vi "复材超声C扫缺陷分析评定软件-用于参考.vi"() -> ()   [LabVIEW 2018]
doc: "使用该模板构建用户界面事件处理设计模式。将模板应用于对话框及其它用户界面。用户也可创建并执行VI可按照与用户界面事件相同方式处理的用户定义事件。"
uses:
  <vilib>/vision/NI_Vision_Development_Module.lvlib
panel:
  out "辅助缺陷评定结果":cluster{dbl, dbl, dbl, dbl, dbl, dbl[][]}
  out "产品规格":cluster{"产品长度（周长）（mm）":dbl, "产品宽度（母线长）（mm）":dbl}
  out "Image Path":path
  out "图像分辨率":T1
  out "Source Image Pixels (U8)":u8[][](array[numeric])
  out "直方图":T2(graph)
  in  "生成原始记录":bool
  in  "去除标注信息":bool caption="缺陷评定"
  in  "缺陷分析及评定":bool caption="辅助定性分析"
  in  "缺陷测量及标注":bool caption="定量分析"
  in  "自定义色彩":bool
  in  "图像处理":bool
  out "Image":T3(plugin-control)
  in  "导入图片":bool
  in  "stop":bool caption="停止"
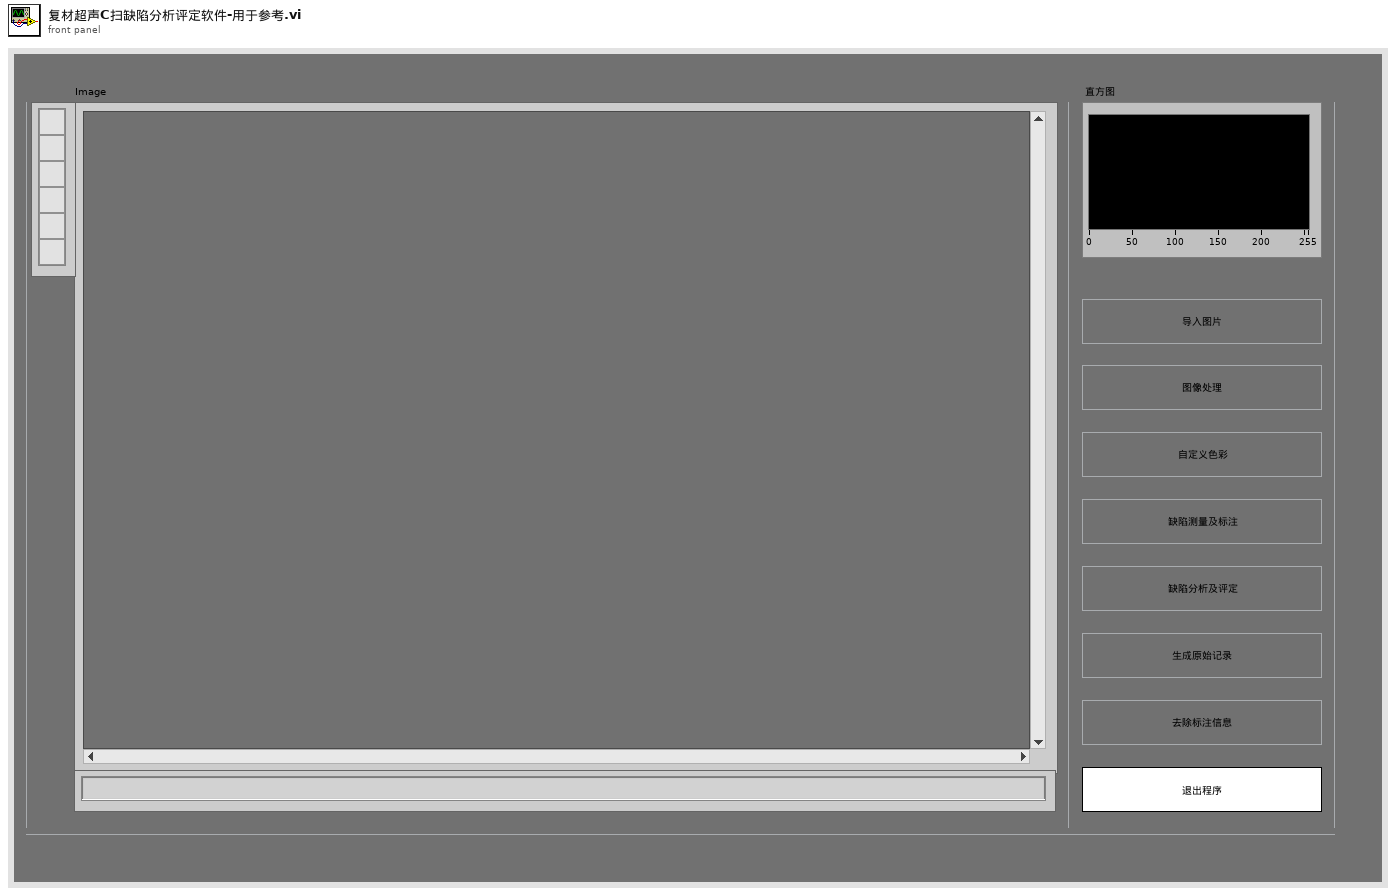
[diagram p1: front panel]
types:
  T1 = cluster{"图像X向分辨率（mm/像素）":dbl, "图像Y向分辨率（mm/像素）":dbl}
  T2 = cluster{"Starting Value":sgl, "Incremental Value":sgl, "Histogram":u32[]}
  T3 = typedef "IMAQ Image.ctl" = refnum<image>
  T4 = cluster{"Zoom Tool":bool, "Selection Tool":bool, "Pan Tool":bool, "Point Tool":bool, "Line Tool":bool, "Rectangle Tool":bool, "Rotated Rectangle Tool":bool, "Polyline Tool":bool, "Polygon Tool":bool, "Freehand Tool":bool, "Closed Freehand Tool":bool, "Ellipse Tool":bool, "Annulus Tool":bool}
  T5 = enum32{"Invalid", "Standard", "Closed", "Hidden", "Minimized", "Maximized"}
  T6 = enum32{"Linear", "Log", "Exp", "Square", "Square root", "Power X", "Power 1/X"}
  T7 = enum32{"Gray", "Binary", "Gradient", "Rainbow", "Temperature"}
  T8 = cluster{"Font Name":string, "Size":i16, "Strikeout?":bool, "Italic?":bool, "Underline?":bool, "Outline?":bool, "Shadow?":bool, "Bold?":bool, "Rotation Angle":dbl}
  T9 = cluster{"Desired Font (Application)":enum16{"User-specified Font", "Application Font", "System Font", "Dialog Font"}, "[User-specified Font]":cluster{"Font Name":string, "Size":i16, "Strikeout?":bool, "Italic?":bool, "Underline?":bool, "Outline?":bool, "Shadow?":bool, "Bold?":bool, "Rotation Angle":dbl}, "Horizontal Alignment":i16, "Vertical Alignment":i16}
  T10 = typedef "Image Type" = u32
  T11 = typedef "imagedata.ctl" = cluster{"image type":i32, "image depth":i32, "image":u8[], "mask":u8[], "colors":u32[], "Rectangle":cluster{"left":i16, "top":i16, "right":i16, "bottom":i16}}
  T12 = cluster{"Red (or Hue) value":u8, "Green (or Sat) value":u8, "Blue (or Light or Val) value":u8}[]
  T13 = typedef "IMAQ Rectangle" = cluster{"Left":i32, "Top":i32, "Right":i32, "Bottom":i32, "Rotation":dbl}
  T14 = typedef "ROI Descriptor" = cluster{"Global Rectangle":i32[], "Contours":cluster{"ID":enum32{"External", "Internal"}, "Type":u32, "Coordinates":i32[]}[]}
  T15 = cluster{"X左上":i32, "Y左上":i32, "X右上":i32, "Y右上":i32, "X左下":i32, "Y左下":i32, "X右下":i32, "Y右下":i32}
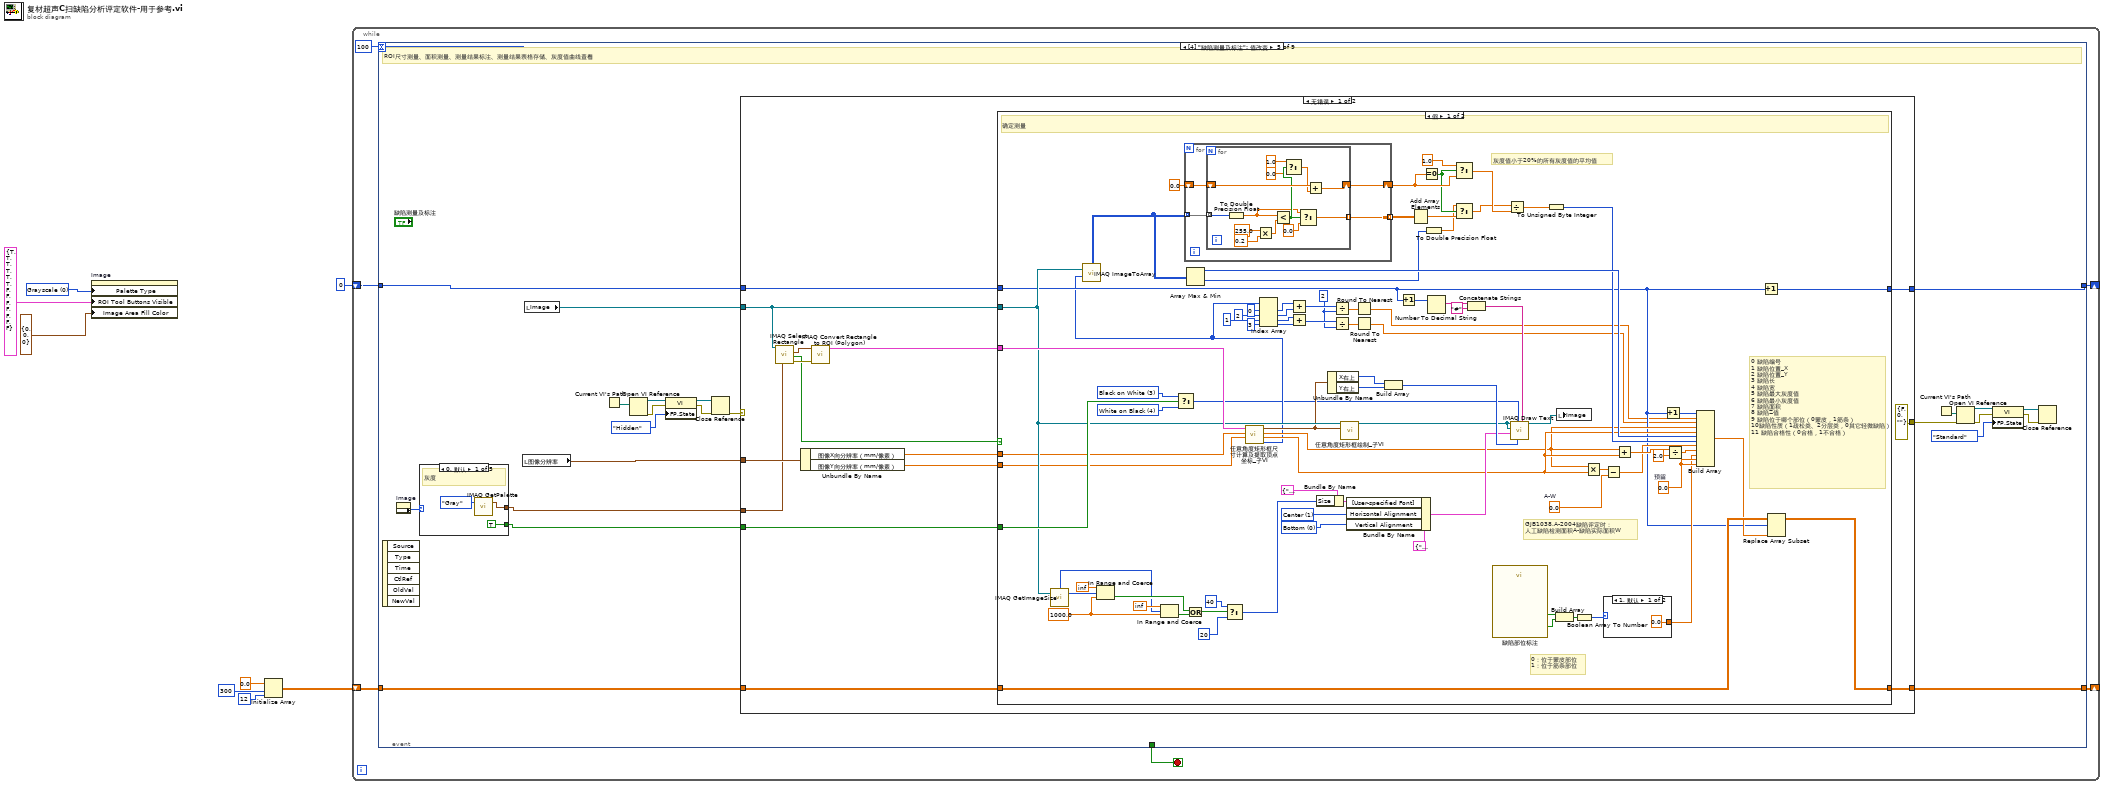
[diagram p0: block diagram]
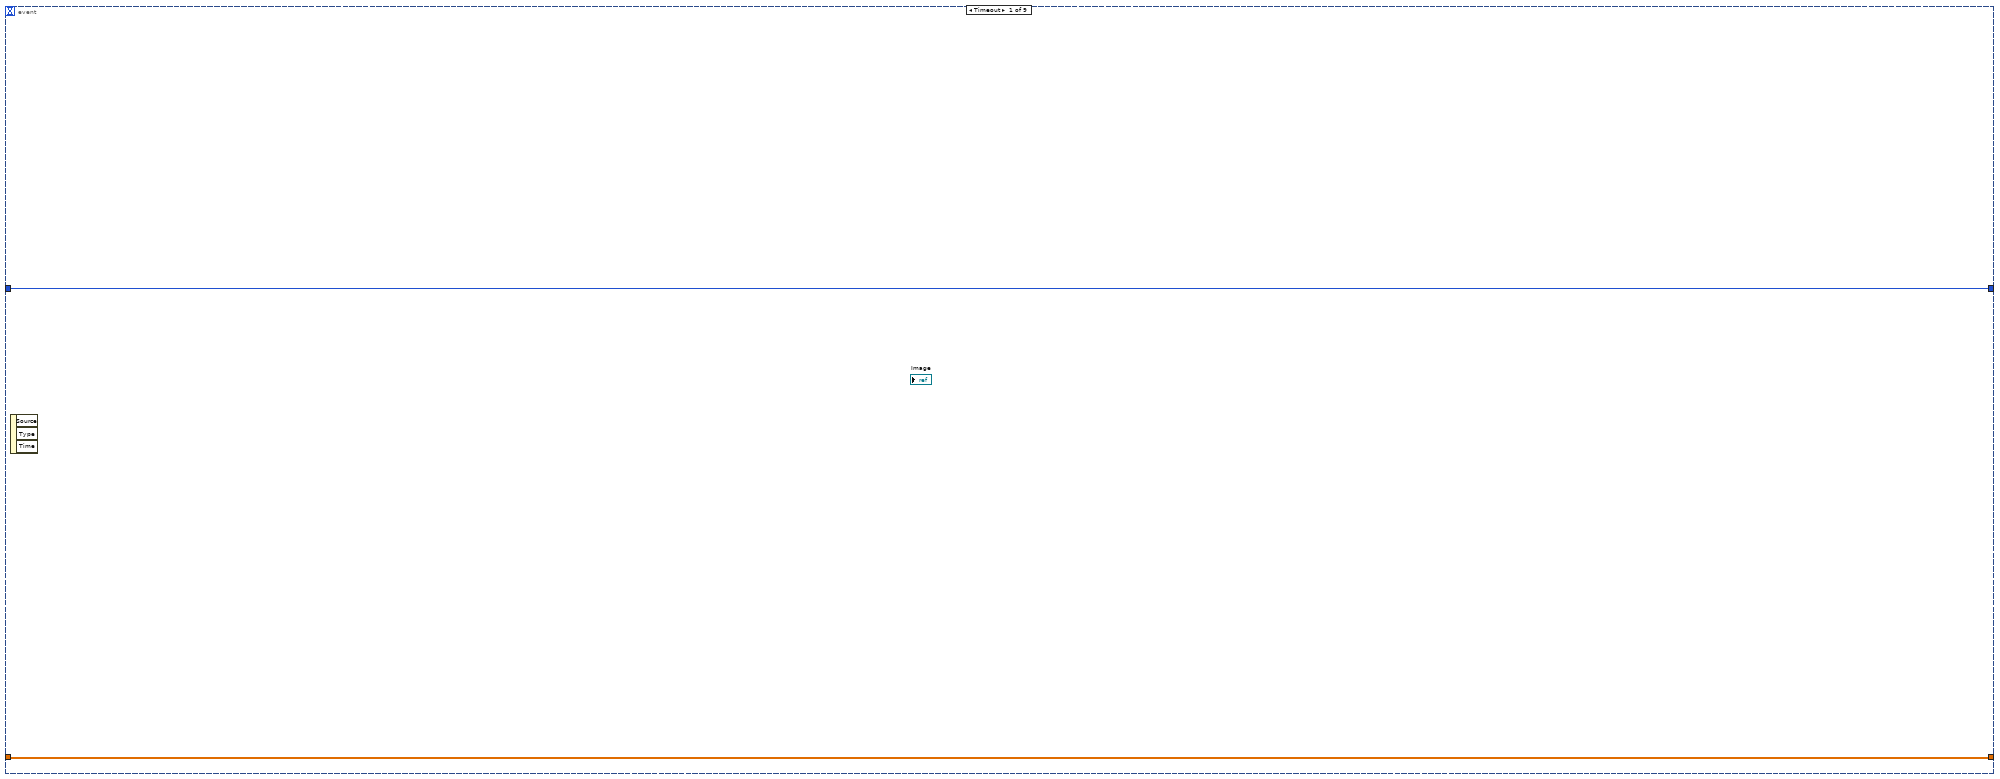
[diagram p2: hidden frame]
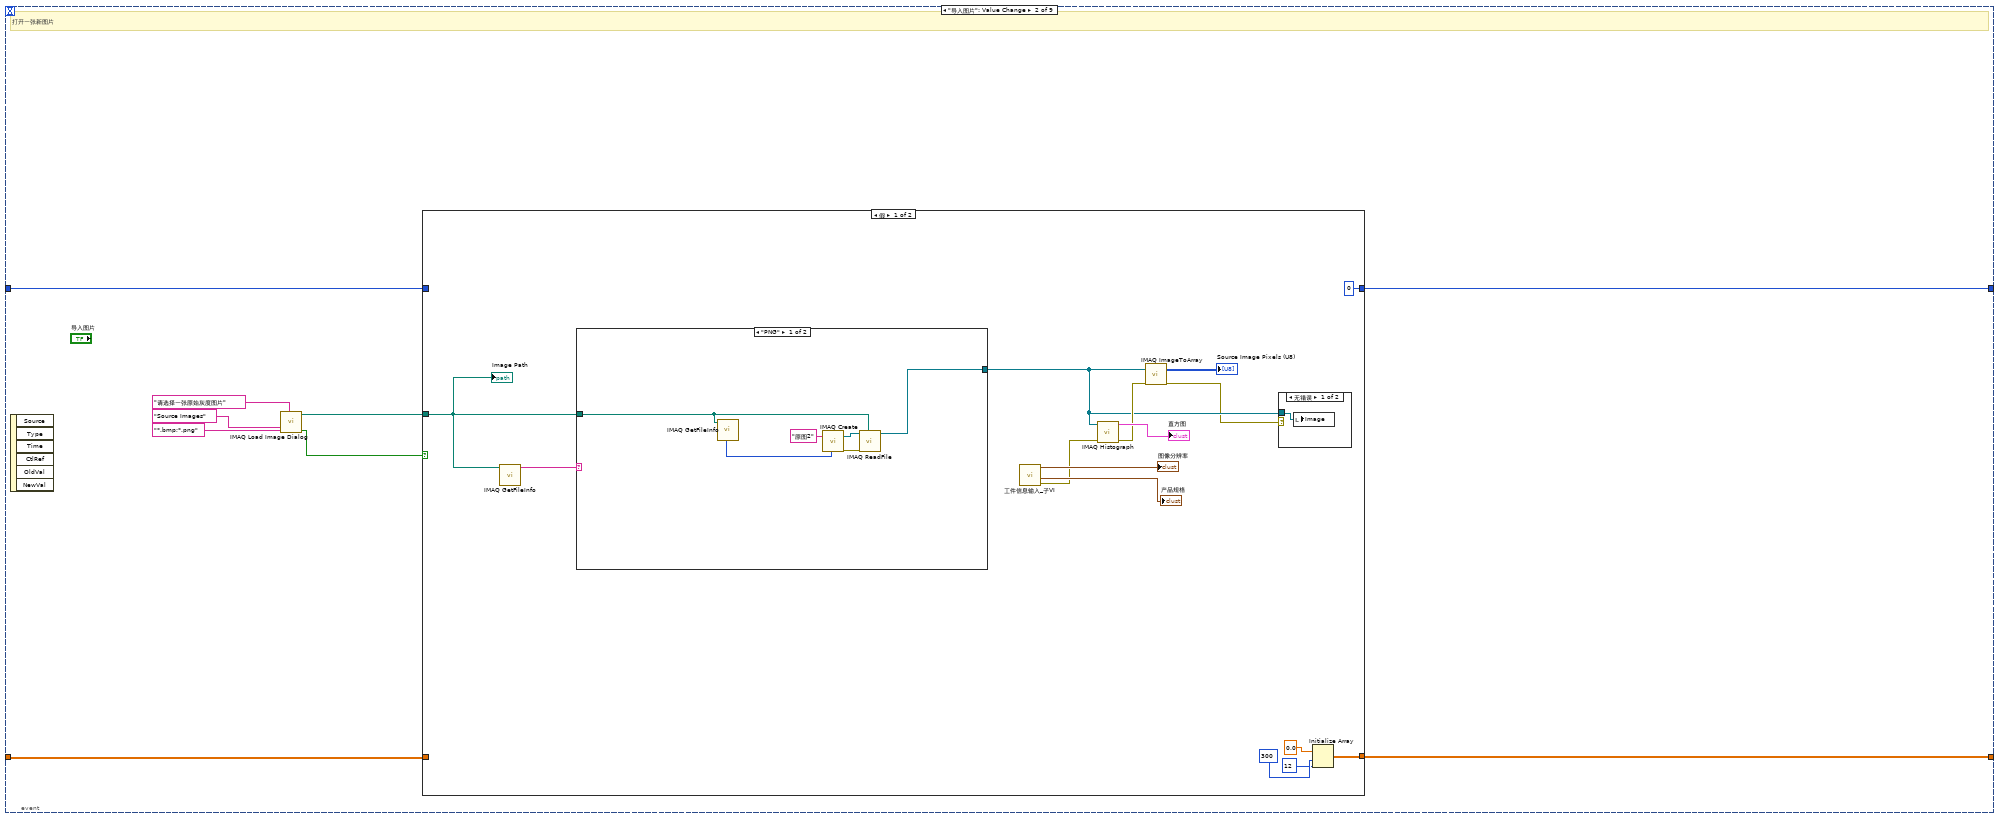
[diagram p3: hidden frame]
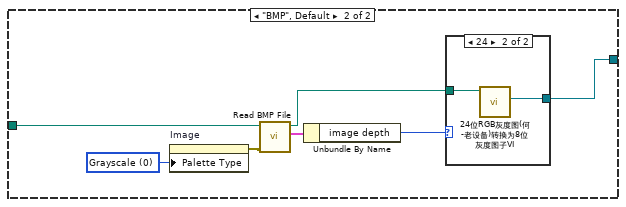
[diagram p5: hidden frame]
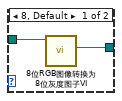
[diagram p6: hidden frame]
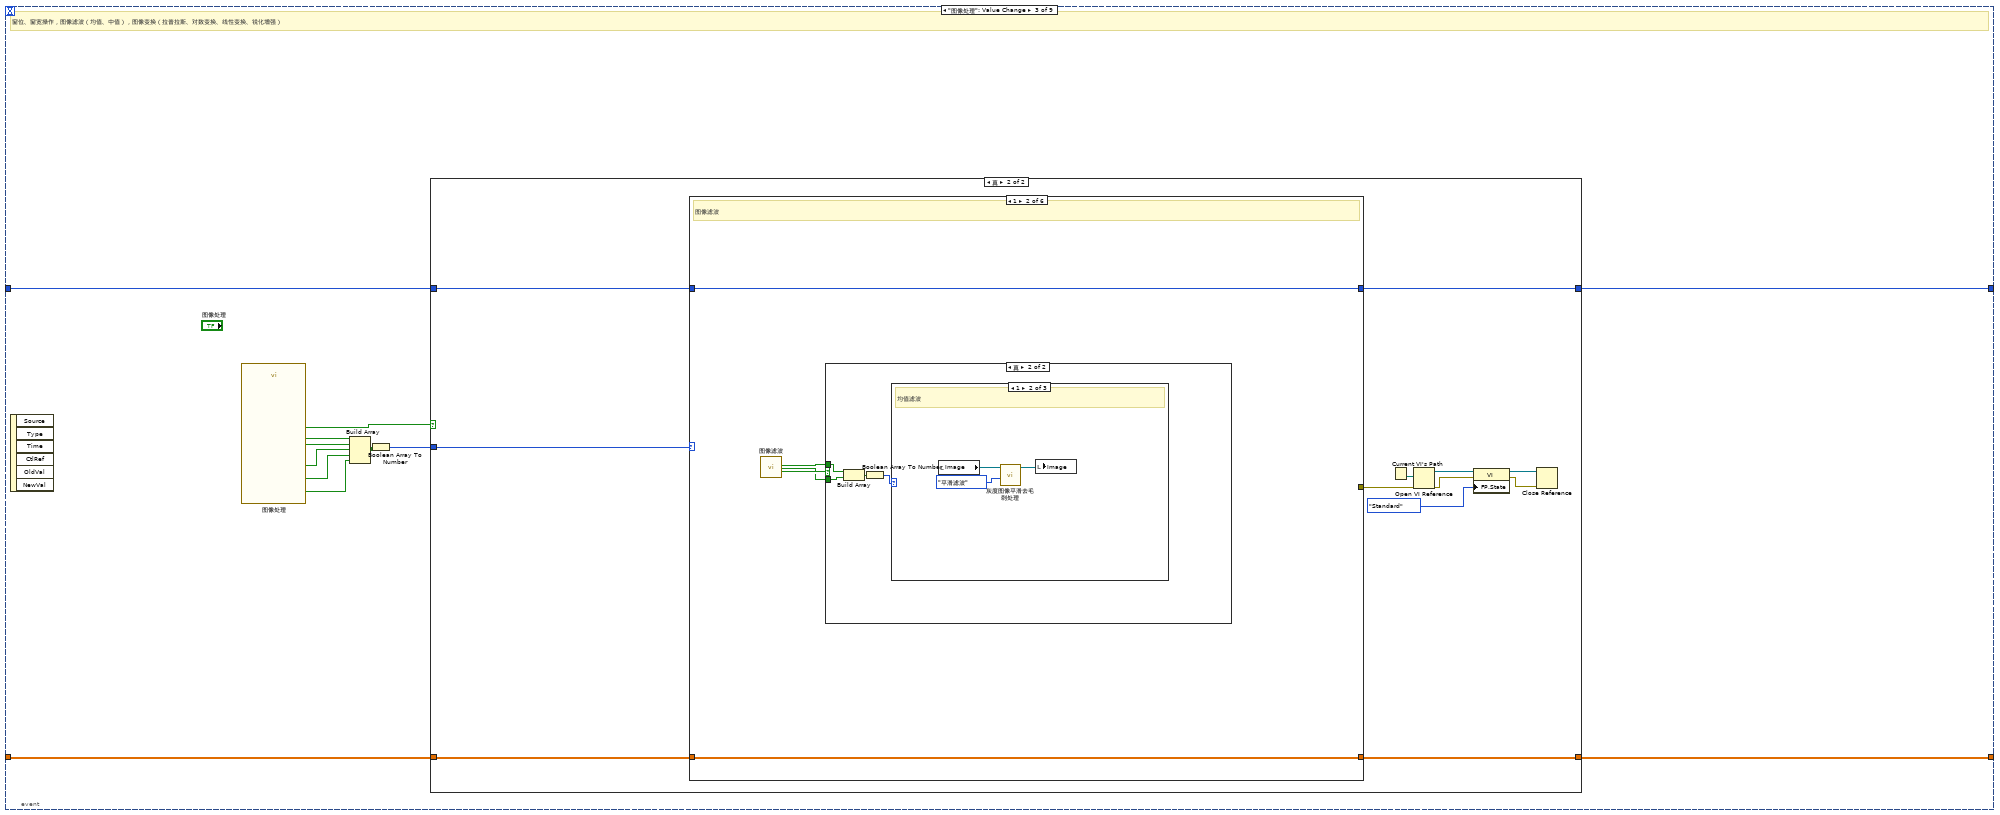
[diagram p8: hidden frame]
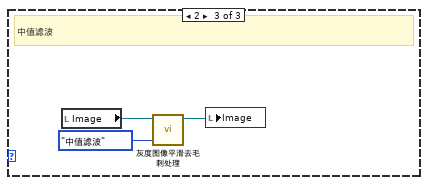
[diagram p13: hidden frame]
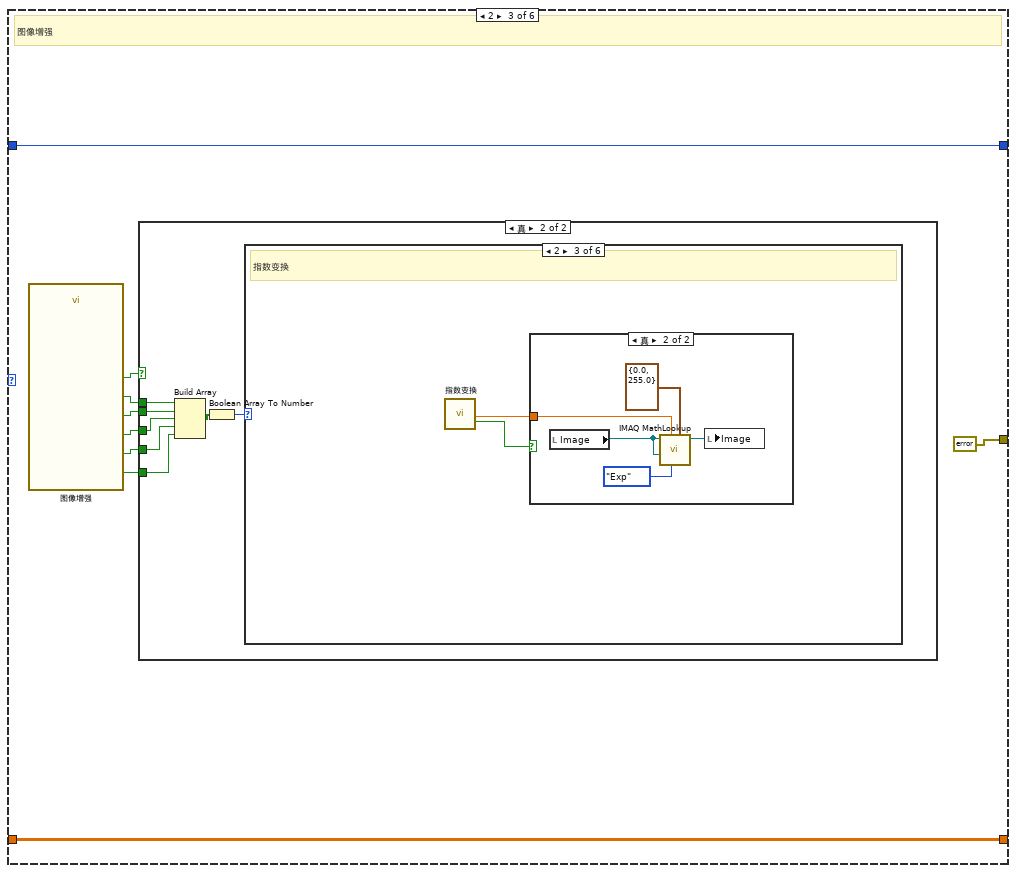
[diagram p14: hidden frame]
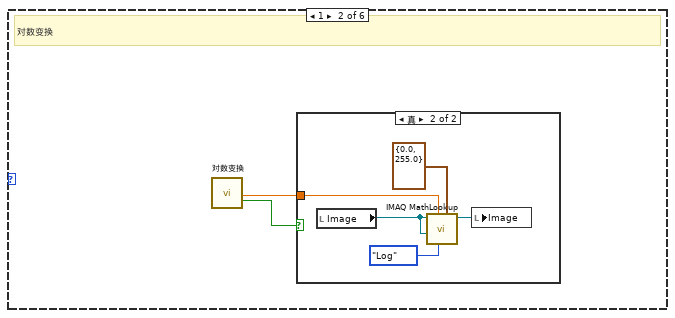
[diagram p17: hidden frame]
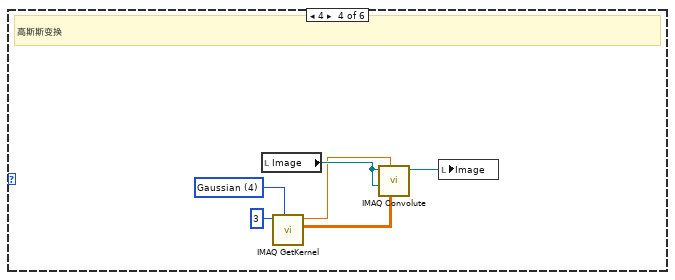
[diagram p20: hidden frame]
diagram:
  w3 = u32 0 items=["Grayscale", "Binary", "Gradient", "Rainbow", "Temperature", "User Defined", "Binary 16 Bit", "Gradient 16 Bit", "Rainbow 16 Bit", "Temperature 16 Bit", "User Defined 16 Bit"] ("Palette:Palette Type")
  n1 = property on="Image" class="ImageControl"("Palette Type"=w3, "ROI Tool Buttons Visible"=T4 {"Zoom Tool"=TRUE, "Selection Tool"=TRUE, "Pan Tool"=TRUE, "Point Tool"=TRUE, "Line Tool"=TRUE, "Rectangle Tool"=TRUE, "Rotated Rectangle Tool"=FALSE, "Polyline Tool"=FALSE, "Polygon Tool"=FALSE, "Freehand Tool"=FALSE, "Closed Freehand Tool"=FALSE, "Ellipse Tool"=FALSE, "Annulus Tool"=FALSE} ("ROI Tool Buttons Visible:All Elements"), "Image Area Fill Color"=cluster{"Red":u8, "Green":u8, "Blue":u8} {"Red"=0, "Green"=0, "Blue"=0} ("Image Area:Background:Fill Color")) -> ()  [unwired: 2 in, 2 out]
  n2 = Initialize Array(0.0 ("元素"), 300 ("维数大小"), 12 ("维数大小")) -> (w6:dbl[][])
  n3 = while {
    shift-right: [w11] -> _
    shift-left: 0 -> [w12]
    shift-right: [w10] -> _
    shift-left: w6 -> [w9]
    stop <- w14 stop-if-true
    n4 = event shown="[4] \"缺陷测量及标注\": 值改变" {
      selector: _ -> [_ _ _ _ _ _ _ _ _]
      dyn-events: _ -> [_ _ _ _ _ _ _ _ _]
      timeout: 100 -> [_ _ _ _ _ _ _ _ _]
      tunnel: [_ _ _ _ _ _ _ _ w668] -> w14
      tunnel: w12 -> [w16 w17 w64 w215 w248 w397 _ w567 _]
      tunnel: [w16 w18 w63 w215 w247 w397 0 w567 0] -> w11
      tunnel: [w15 w20 w62 w207 w246 w395 w515 w527 dbl[][] []] -> w10
      tunnel: w9 -> [w15 w19 w61 w207 w236 w396 _ w527 _]
      event Timeout {
        n5 = event-data() -> ()  [unwired: 1 in, 3 out]
      }
      event "导入图片": Value Change {
        # "打开一张新图片"
        n6 = event-data() -> ()  [unwired: 1 in, 6 out]
        n7 = call "IMAQ Load Image Dialog"("Pattern Label"="Source Images", "Prompt"="请选择一张原始灰度图片" ("prompt"), "Pattern"="*.bmp;*.png") -> ("Cancelled?"=w21:bool, "Path"=w23:path)  [unwired: 6 in, 1 out]
        n8 = case shown="假" w21 {
          tunnel: w23 -> [w35 _]
          tunnel: [w27 w60] -> w20
          tunnel: w19 -> [_ w60]
          tunnel: [0 w59] -> w18
          tunnel: w17 -> [_ w59]
          frame False {
            n9 = call "IMAQ GetFileInfo"("File Path"=w35) -> ("File Type"=w40:string)  [unwired: 4 in, 6 out]
            n10 = case shown="\"PNG\"" w40 {
              tunnel: w35 -> [w43 w54]
              tunnel: [w42 w53] -> w36
              frame "PNG" {
                n11 = call "IMAQ GetFileInfo"("File Path"=w43) -> ("Image Type"=w45:T10)  [unwired: 4 in, 6 out]
                n12 = call "IMAQ Create"("Image Name"="原图2", "Image Type"=w45) -> ("New Image"=w46:T3, "error out"=w47:errorcluster)  [unwired: 3 in]
                n13 = call "IMAQ ReadFile"("File Path"=w43, "error in (no error)"=w47, "Image"=w46) -> ("Image Out"=w42:T3)  [unwired: 4 in, 4 out]
              }
              frame "BMP", Default {
                w49 = u32 0 items=["Grayscale", "Binary", "Gradient", "Rainbow", "Temperature", "User Defined", "Binary 16 Bit", "Gradient 16 Bit", "Rainbow 16 Bit", "Temperature 16 Bit", "User Defined 16 Bit"] ("Palette:Palette Type")
                n14 = property on="Image" class="ImageControl"("Palette Type"=w49) -> (error out=w48:errorcluster)  [unwired: 2 in, 1 out]
                n15 = call <vilib>:"Read BMP File.vi"("error in (no error)"=w48, "path to BMP file"=w54) -> ("image data"=w52:T11, "path"=w50:path)  [unwired: 7 in, 1 out]
                n16 = Unbundle By Name(w52) -> ("image depth"=w51:i32)
                n17 = case shown="24" w51 {
                  tunnel: w50 -> [w56 w58]
                  tunnel: [w55 w57] -> w53
                  frame 8, Default {
                    n18 = call "8位RGB图像转换为8位灰度图子VI.vi"("path to BMP file"=w56) -> ("转换后的原始图像"=w55:T3)  [unwired: 8 in, 2 out]
                  }
                  frame 24 {
                    n19 = call "24位RGB灰度图(何-老设备)转换为8位灰度图子VI.vi"("File Path"=w58) -> ("转换后的原始图像"=w57:T3)  [unwired: 8 in, 2 out]
                  }
                }
              }
            }
            n20 = call "工件信息输入_子VI.vi"() -> ("错误常量out"=w31:errorcluster, "产品规格"=→"产品规格":cluster{"产品长度（周长）（mm）":dbl, "产品宽度（母线长）（mm）":dbl}, "图像分辨率"=→"图像分辨率":T1)  [unwired: 9 in]
            n21 = call "IMAQ Histograph"("error in (no error)"=w31, "Image"=w36) -> ("error out"=w37:errorcluster, "Histogram Graph"=→"直方图":T2)  [unwired: 6 in, 2 out]
            n22 = call "IMAQ ImageToArray"("error in (no error)"=w37, "Image"=w36) -> ("error out"=w34:errorcluster, "Image Pixels (U8)"=→"Source Image Pixels (U8)":u8[][])  [unwired: 2 in, 3 out]
            n23 = case shown="无错误" w34 {
              tunnel: w36 -> [w41 _]
              frame No Error {
                n24 = local write "Image"(w41) -> ()
              }
              frame Error {
              }
            }
            n25 = Initialize Array(0.0 ("元素"), 300 ("维数大小"), 12 ("维数大小")) -> (w27:dbl[][])
            "Image Path" <- w35
          }
          frame True {
          }
        }
      }
      event "图像处理": Value Change {
        # "窗位、窗宽操作，图像滤波（均值、中值），图像变换（拉普拉斯、对数变换、线性变换、锐化增强）"
        n26 = event-data() -> ()  [unwired: 1 in, 6 out]
        n27 = call "图像处理"() -> ("撤销图像处理"=w65:bool, "线性灰度值测量"=w66:bool, "窗位窗宽"=w71:bool, "图像增强"=w67:bool, "图像滤波"=w72:bool, "确定"=w68:bool)  [unwired: 13 in, 1 out]
        n28 = Build Array(w72, w67, w71, w66, w65) -> (w70:bool[])
        n29 = Boolean Array To Number(Boolean array=w70) -> (number=w69:u32)
        n30 = case shown="真" w68 {
          tunnel: w69 -> [_ w86]
          tunnel: w64 -> [w73 w78]
          tunnel: [w73 w77] -> w63
          tunnel: [w74 w76] -> w62
          tunnel: w61 -> [w74 w75]
          frame False {
          }
          frame True {
            n31 = case shown="1" w86 {
              tunnel: [_ _ errorcluster {"status"=FALSE, "code"=0, "source"=""} ("错误输入（无错误）") _ _ _] -> w79
              tunnel: w78 -> [w88 w89 w105 w155 w180 w201]
              tunnel: [w88 w89 w105 w155 w180 w201] -> w77
              tunnel: [w87 w90 w104 w154 w179 w202] -> w76
              tunnel: w75 -> [w87 w90 w104 w154 w179 w202]
              frame 0, Default {
              }
              frame 1 {
                # "图像滤波"
                n32 = call "图像滤波"() -> ("均值滤波"=w92:bool, "中值滤波"=w91:bool, "确定"=w93:bool)  [unwired: 16 in, 1 out]
                n33 = case shown="真" w93 {
                  tunnel: w92 -> [_ w96]
                  tunnel: w91 -> [_ w95]
                  frame False {
                  }
                  frame True {
                    n34 = Build Array(w96, w95) -> (w97:bool[])
                    n35 = Boolean Array To Number(Boolean array=w97) -> (number=w94:u32)
                    n36 = case shown="1" w94 {
                      frame 0, Default {
                      }
                      frame 1 {
                        # "均值滤波"
                        n37 = local read "Image"() -> (w100:T3)
                        n38 = call "灰度图像平滑去毛刺处理.vi"("滤波方法选择"=enum16{"中值滤波", "平滑滤波"}."平滑滤波", "Image"=w100) -> ("Image Out"=w99:T3)  [unwired: 9 in]
                        n39 = local write "Image"(w99) -> ()
                      }
                      frame 2 {
                        # "中值滤波"
                        n40 = local read "Image"() -> (w103:T3)
                        n41 = call "灰度图像平滑去毛刺处理.vi"("滤波方法选择"=enum16{"中值滤波", "平滑滤波"}."中值滤波", "Image"=w103) -> ("Image Out"=w102:T3)  [unwired: 9 in]
                        n42 = local write "Image"(w102) -> ()
                      }
                    }
                  }
                }
              }
              frame 2 {
                # "图像增强"
                n43 = call "图像增强"() -> ("幂变换"=w107:bool, "阈值变换"=w108:bool, "高斯变换"=w109:bool, "指数变换"=w110:bool, "对数变换"=w111:bool, "确定"=w112:bool)  [unwired: 13 in, 1 out]
                n44 = case shown="真" w112 {
                  tunnel: w111 -> [_ w117]
                  tunnel: w110 -> [_ w116]
                  tunnel: w109 -> [_ w115]
                  tunnel: w108 -> [_ w114]
                  tunnel: w107 -> [_ w113]
                  frame False {
                  }
                  frame True {
                    n45 = Build Array(w117, w116, w115, w114, w113) -> (w119:bool[])
                    n46 = Boolean Array To Number(Boolean array=w119) -> (number=w118:u32)
                    n47 = case shown="2" w118 {
                      frame 0, Default {
                      }
                      frame 1 {
                        # "对数变换"
                        n48 = call "对数变换"() -> ("变换系数K"=w120:dbl, "确定"=w121:bool)  [unwired: 17 in, 1 out]
                        n49 = case shown="真" w121 {
                          tunnel: w120 -> [_ w122]
                          frame False {
                          }
                          frame True {
                            n50 = local read "Image"() -> (w126:T3)
                            n51 = call "IMAQ MathLookup"("Range"=cluster{"Minimum":sgl, "Maximum":sgl} {"Minimum"=0.0, "Maximum"=255.0}, "Operator"=T6."Log", "X Value"=w122, "Image Dst"=w126, "Image Src"=w126) -> ("Image Dst Out"=w124:T3)  [unwired: 5 in, 1 out]
                            n52 = local write "Image"(w124) -> ()
                          }
                        }
                      }
                      frame 2 {
                        # "指数变换"
                        n53 = call "指数变换"() -> ("变换系数K"=w127:dbl, "确定"=w128:bool)  [unwired: 17 in, 1 out]
                        n54 = case shown="真" w128 {
                          tunnel: w127 -> [_ w129]
                          frame False {
                          }
                          frame True {
                            n55 = local read "Image"() -> (w133:T3)
                            n56 = call "IMAQ MathLookup"("Range"=cluster{"Minimum":sgl, "Maximum":sgl} {"Minimum"=0.0, "Maximum"=255.0}, "Operator"=T6."Exp", "X Value"=w129, "Image Dst"=w133, "Image Src"=w133) -> ("Image Dst Out"=w131:T3)  [unwired: 5 in, 1 out]
                            n57 = local write "Image"(w131) -> ()
                          }
                        }
                      }
                      frame 4 {
                        w139 = u16 4 items=["Gradient"=1, "Laplacian"=2, "Smoothing"=3, "Gaussian"=4] ("Kernel Family")
                        # "高斯斯变换"
                        n58 = local read "Image"() -> (w136:T3)
                        n59 = call "IMAQ GetKernel"("Kernel Family"=w139, "Kernel Size (3,5,...)"=3) -> ("Kernel"=w137:sgl[][], "Divider"=w134:sgl)  [unwired: 6 in, 2 out]
                        n60 = call "IMAQ Convolute"("Kernel"=w137, "Divider (kernel sum)"=w134, "Image Dst"=w136, "Image Src"=w136) -> ("Image Dst Out"=w135:T3)  [unwired: 6 in, 1 out]
                        n61 = local write "Image"(w135) -> ()
                      }
                      frame 8 {
                        # "阈值变换"
                        n62 = call "阈值范围选择子VI.vi"() -> ("阈值范围"=w140:cluster{"Lower value":sgl, "Upper value":sgl}, "确定执行"=w141:bool)  [unwired: 10 in]
                        n63 = case shown="真" w141 {
                          tunnel: w140 -> [_ w143]
                          frame False {
                          }
                          frame True {
                            n64 = local read "Image"() -> (w146:T3)
                            n65 = call "IMAQ Threshold"("Replace Value"=sgl 255.0, "Keep/Replace Value (Replace)"=TRUE, "Range"=w143, "Image Dst"=w146, "Image Src"=w146) -> ("Image Dst Out"=w145:T3)  [unwired: 5 in, 1 out]
                            n66 = local write "Image"(w145) -> ()
                          }
                        }
                      }
                      frame 16 {
                        # "幂变换"
                        n67 = call "幂变换"() -> ("变换系数K"=w147:dbl, "确定"=w148:bool)  [unwired: 17 in, 1 out]
                        n68 = case shown="真" w148 {
                          tunnel: w147 -> [_ w149]
                          frame False {
                          }
                          frame True {
                            n69 = local read "Image"() -> (w153:T3)
                            n70 = call "IMAQ MathLookup"("Range"=cluster{"Minimum":sgl, "Maximum":sgl} {"Minimum"=0.0, "Maximum"=255.0}, "Operator"=T6."Power 1/X", "X Value"=w149, "Image Dst"=w153, "Image Src"=w153) -> ("Image Dst Out"=w151:T3)  [unwired: 5 in, 1 out]
                            n71 = local write "Image"(w151) -> ()
                          }
                        }
                      }
                    }
                  }
                }
              }
              frame 4 {
                # "窗位窗宽"
                n72 = Two Button Dialog(message="确定进行窗位窗宽操作？" ("消息")) -> (T button?=w157:bool)  [unwired: 2 in]
                n73 = case shown="真" w157 {
                  frame False {
                  }
                  frame True {
                    n74 = property on="Image" class="ImageControl"() -> (error out=w159:errorcluster, "Palette Type"=w166:u32)  [unwired: 2 in, 1 out]
                    n75 = Current VI's Path() -> (path=w161:path)
                    n76 = Open VI Reference(vi path=w161, error in (no error)=w159) -> (vi reference=w162:refnum<vi>, error out=w164:errorcluster)  [unwired: 4 in]
                    n77 = case shown="4" w166 {
                      tunnel: [w170 w172 w174 w176 w178] -> w167
                      frame 0, Default {
                        # "灰度"
                        n78 = call "IMAQ GetPalette"("Palette Number (gray)"=T7."Gray") -> ("Color Palette"=w170:cluster{"Red":u8, "Green":u8, "Blue":u8}[])  [unwired: 4 in, 1 out]
                      }
                      frame 2 {
                        # "梯度"
                        n79 = call "IMAQ GetPalette"("Palette Number (gray)"=T7."Gradient") -> ("Color Palette"=w172:cluster{"Red":u8, "Green":u8, "Blue":u8}[])  [unwired: 4 in, 1 out]
                      }
                      frame 3 {
                        # "彩虹"
                        n80 = call "IMAQ GetPalette"("Palette Number (gray)"=T7."Rainbow") -> ("Color Palette"=w174:cluster{"Red":u8, "Green":u8, "Blue":u8}[])  [unwired: 4 in, 1 out]
                      }
                      frame 4 {
                        # "温度"
                        n81 = call "IMAQ GetPalette"("Palette Number (gray)"=T7."Temperature") -> ("Color Palette"=w176:cluster{"Red":u8, "Green":u8, "Blue":u8}[])  [unwired: 4 in, 1 out]
                      }
                      frame 5 {
                        # "自定义"
                        n82 = property on="Image" class="ImageControl"() -> ("User Palette"=w178:cluster{"Red":u8, "Green":u8, "Blue":u8}[])  [unwired: 2 in, 2 out]
                      }
                    }
                    n83 = property class="VI"(reference=w162, error in=w164, "FP.State"=T5."Hidden" ("前面板窗口:状态")) -> (reference out=w163:refnum<vi>, error out=w165:errorcluster)
                    n84 = local read "Source Image Pixels (U8)"() -> (w168:u8[][])
                    n85 = Close Reference(reference=w163, error in (no error)=w165) -> ()  [unwired: 1 out]
                    n86 = local read "Image"() -> (w158:T3)
                    n87 = call "窗位窗宽调整子VI.vi"("Image in"=w158, "Palette:User Palette"=w167, "Palette:Palette Type"=w166, "Image Pixels (U8)"=w168) -> ("Image out"=w169:T3)  [unwired: 7 in]
                    n88 = local write "Image"(w169) -> ()
                  }
                }
              }
              frame 8 {
                # "查看线灰度值曲线，用于精确测量"
                n89 = Current VI's Path() -> (path=w187:path)
                n90 = Open VI Reference(vi path=w187) -> (vi reference=w186:refnum<vi>, error out=w184:errorcluster)  [unwired: 5 in]
                n91 = property class="VI"(reference=w186, error in=w184, "FP.State"=T5."Hidden" ("前面板窗口:状态")) -> (reference out=w185:refnum<vi>, error out=w183:errorcluster)
                n92 = Close Reference(reference=w185, error in (no error)=w183) -> (error out=w181:errorcluster)
                n93 = case shown="无错误" w181 {
                  frame No Error {
                    n94 = property on="Image" class="ImageControl"() -> ("Palette Type"=w189:u32)  [unwired: 2 in, 2 out]
                    n95 = case shown="2" w189 {
                      tunnel: [w192 w194 w196 w198 w200] -> w188
                      frame 0, Default {
                        # "灰度"
                        n96 = call "IMAQ GetPalette"("Palette Number (gray)"=T7."Gray") -> ("Color Palette"=w192:cluster{"Red":u8, "Green":u8, "Blue":u8}[])  [unwired: 4 in, 1 out]
                      }
                      frame 2 {
                        # "梯度"
                        n97 = call "IMAQ GetPalette"("Palette Number (gray)"=T7."Gradient") -> ("Color Palette"=w194:cluster{"Red":u8, "Green":u8, "Blue":u8}[])  [unwired: 4 in, 1 out]
                      }
                      frame 3 {
                        # "彩虹"
                        n98 = call "IMAQ GetPalette"("Palette Number (gray)"=T7."Rainbow") -> ("Color Palette"=w196:cluster{"Red":u8, "Green":u8, "Blue":u8}[])  [unwired: 4 in, 1 out]
                      }
                      frame 4 {
                        # "温度"
                        n99 = call "IMAQ GetPalette"("Palette Number (gray)"=T7."Temperature") -> ("Color Palette"=w198:cluster{"Red":u8, "Green":u8, "Blue":u8}[])  [unwired: 4 in, 1 out]
                      }
                      frame 5 {
                        # "自定义"
                        n100 = property on="Image" class="ImageControl"() -> ("User Palette"=w200:cluster{"Red":u8, "Green":u8, "Blue":u8}[])  [unwired: 2 in, 2 out]
                      }
                    }
                    n101 = local read "Image"() -> (w191:T3)
                    n102 = local read "图像分辨率"() -> (w190:T1)
                    n103 = call "线性灰度值曲线查看子VI.vi"("Palette:User Palette"=w188, "图像分辨率"=w190, "Image"=w191) -> ()  [unwired: 9 in]
                  }
                  frame Error {
                  }
                }
              }
              frame 16 {
                # "撤销图像处理，恢复原图"
                n104 = local read "Source Image Pixels (U8)"() -> (w206:u8[][])
                n105 = call "IMAQ Create"("Image Name"="P1") -> ("New Image"=w205:T3)  [unwired: 4 in, 1 out]
                n106 = call "IMAQ ArrayToImage"("Image Pixels (U8)"=w206, "Image"=w205) -> ("Image Out"=w204:T3)  [unwired: 8 in, 1 out]
                n107 = local write "Image"(w204) -> ()
              }
            }
            n108 = Current VI's Path() -> (path=w85:path)
            n109 = Open VI Reference(vi path=w85, error in (no error)=w79) -> (vi reference=w84:refnum<vi>, error out=w81:errorcluster)  [unwired: 4 in]
            n110 = property class="VI"(reference=w84, error in=w81, "FP.State"=T5."Standard" ("前面板窗口:状态")) -> (reference out=w82:refnum<vi>, error out=w80:errorcluster)
            n111 = Close Reference(reference=w82, error in (no error)=w80) -> ()  [unwired: 1 out]
          }
        }
      }
      event "自定义色彩": Value Change {
        # "色彩、色阶自定义"
        n112 = event-data() -> ()  [unwired: 1 in, 6 out]
        n113 = call "调色板"() -> ("自定义显示"=w209:bool, "温度显示"=w210:bool, "彩虹显示"=w211:bool, "梯度显示"=w212:bool, "灰度显示"=w213:bool, "确定"=w214:bool)  [unwired: 13 in, 1 out]
        n114 = Build Array(w213, w212, w211, w210, w209) -> (w208:bool[])
        n115 = case shown="真" w214 {
          tunnel: w208 -> [_ w218]
          frame False {
          }
          frame True {
            n116 = Boolean Array To Number(Boolean array=w218) -> (number=w217:u32)
            n117 = case shown="16" w217 {
              tunnel: [w219 w220 w221 w222 w223 w225] -> w216
              frame 0, Default {
                w219 = u32 0 items=["Grayscale", "Binary", "Gradient", "Rainbow", "Temperature", "User Defined", "Binary 16 Bit", "Gradient 16 Bit", "Rainbow 16 Bit", "Temperature 16 Bit", "User Defined 16 Bit"] ("Palette:Palette Type")
              }
              frame 1 {
                w220 = u32 0 items=["Grayscale", "Binary", "Gradient", "Rainbow", "Temperature", "User Defined", "Binary 16 Bit", "Gradient 16 Bit", "Rainbow 16 Bit", "Temperature 16 Bit", "User Defined 16 Bit"] ("Palette:Palette Type")
                # "灰度"
              }
              frame 2 {
                w221 = u32 2 items=["Grayscale", "Binary", "Gradient", "Rainbow", "Temperature", "User Defined", "Binary 16 Bit", "Gradient 16 Bit", "Rainbow 16 Bit", "Temperature 16 Bit", "User Defined 16 Bit"] ("Palette:Palette Type")
                # "梯度"
              }
              frame 4 {
                w222 = u32 3 items=["Grayscale", "Binary", "Gradient", "Rainbow", "Temperature", "User Defined", "Binary 16 Bit", "Gradient 16 Bit", "Rainbow 16 Bit", "Temperature 16 Bit", "User Defined 16 Bit"] ("Palette:Palette Type")
                # "彩虹"
              }
              frame 8 {
                w223 = u32 4 items=["Grayscale", "Binary", "Gradient", "Rainbow", "Temperature", "User Defined", "Binary 16 Bit", "Gradient 16 Bit", "Rainbow 16 Bit", "Temperature 16 Bit", "User Defined 16 Bit"] ("Palette:Palette Type")
                # "温度"
              }
              frame 16 {
                w225 = u32 5 items=["Grayscale", "Binary", "Gradient", "Rainbow", "Temperature", "User Defined", "Binary 16 Bit", "Gradient 16 Bit", "Rainbow 16 Bit", "Temperature 16 Bit", "User Defined 16 Bit"] ("Palette:Palette Type")
                # "自定义"
                n118 = call "自定义成像色谱20200214.vi"() -> ("Color palette"=w224:T12)  [unwired: 8 in, 1 out]
                n119 = property on="Image" class="ImageControl"("User Palette"=w224) -> ()  [unwired: 2 in, 2 out]
              }
            }
            n120 = property on="Image" class="ImageControl"("Palette Type"=w216) -> ()  [unwired: 2 in, 2 out]
          }
        }
      }
      event "缺陷测量及标注": Value Change {
        # "ROI尺寸测量、面积测量、测量结果标注、测量结果表格存储、灰度值曲线查看"
        n121 = event-data() -> ()  [unwired: 1 in, 6 out]
        n122 = property on="Image" class="ImageControl"() -> ("Palette Type"=w245:u32)  [unwired: 2 in, 2 out]
        n123 = case shown="0, 默认" w245 {
          tunnel: [w373 w375 w377 w379 w381] -> w244
          tunnel: [TRUE _ _ _ _] -> w237
          frame 0, Default {
            # "灰度"
            n124 = call "IMAQ GetPalette"("Palette Number (gray)"=T7."Gray") -> ("Color Palette"=w373:cluster{"Red":u8, "Green":u8, "Blue":u8}[])  [unwired: 4 in, 1 out]
          }
          frame 2 {
            # "梯度"
            n125 = call "IMAQ GetPalette"("Palette Number (gray)"=T7."Gradient") -> ("Color Palette"=w375:cluster{"Red":u8, "Green":u8, "Blue":u8}[])  [unwired: 4 in, 1 out]
          }
          frame 3 {
            # "彩虹"
            n126 = call "IMAQ GetPalette"("Palette Number (gray)"=T7."Rainbow") -> ("Color Palette"=w377:cluster{"Red":u8, "Green":u8, "Blue":u8}[])  [unwired: 4 in, 1 out]
          }
          frame 4 {
            # "温度"
            n127 = call "IMAQ GetPalette"("Palette Number (gray)"=T7."Temperature") -> ("Color Palette"=w379:cluster{"Red":u8, "Green":u8, "Blue":u8}[])  [unwired: 4 in, 1 out]
          }
          frame 5 {
            # "自定义"
            n128 = property on="Image" class="ImageControl"() -> ("User Palette"=w381:cluster{"Red":u8, "Green":u8, "Blue":u8}[])  [unwired: 2 in, 2 out]
          }
        }
        n129 = local read "图像分辨率"() -> (w234:T1)
        n130 = local read "Image"() -> (w235:T3)
        n131 = Current VI's Path() -> (path=w233:path)
        n132 = Open VI Reference(vi path=w233) -> (vi reference=w232:refnum<vi>, error out=w230:errorcluster)  [unwired: 5 in]
        n133 = property class="VI"(reference=w232, error in=w230, "FP.State"=T5."Hidden" ("前面板窗口:状态")) -> (reference out=w231:refnum<vi>, error out=w229:errorcluster)
        n134 = Close Reference(reference=w231, error in (no error)=w229) -> (error out=w227:errorcluster)
        n135 = case shown="无错误" w227 {
          tunnel: w248 -> [w263 w370]
          tunnel: [w262 w370] -> w247
          tunnel: w235 -> [w253 _]
          tunnel: w234 -> [w261 _]
          tunnel: [w260 w371] -> w246
          tunnel: w236 -> [w259 w371]
          tunnel: w244 -> [w252 _]
          tunnel: w237 -> [w258 _]
          tunnel: [errorcluster {"status"=FALSE, "code"=0, "source"=""} ("error in (no error)") _] -> w226
          frame No Error {
            n136 = call "IMAQ Select Rectangle"("Color Palette"=w252, "Image In"=w253) -> ("error out"=w254:errorcluster, "Cancelled"=w249:bool, "Rectangle"=w255:T13)  [unwired: 6 in, 1 out]
            n137 = Unbundle By Name(w261) -> ("图像X向分辨率（mm/像素）"=w257:dbl, "图像Y向分辨率（mm/像素）"=w256:dbl)
            n138 = call "IMAQ Convert Rectangle to ROI (Polygon)"("error in (no error)"=w254, "Rectangle"=w255) -> ("ROI Descriptor"=w251:T14)  [unwired: 6 in, 2 out]
            n139 = case shown="假" w249 {
              tunnel: w263 -> [w292 w369]
              tunnel: [w348 w369] -> w262
              tunnel: w253 -> [w301 _]
              tunnel: [w340 w368] -> w260
              tunnel: w259 -> [w342 w368]
              tunnel: w251 -> [w302 _]
              tunnel: w258 -> [w314 _]
              tunnel: w257 -> [w300 _]
              tunnel: w256 -> [w299 _]
              frame False {
                w272 = 2 ("y")
                w290 = i16 0 items=["Bottom", "Top", "Baseline"] ("Vertical Alignment")
                w288 = 1000.0 ("下限")
                w312 = 4 items=["White", "Black", "Inverted", "Black on White", "White on Black"] ("Color")
                w328 = 0.0  # A-W
                w336 = 0.0  # 预留
                w313 = 3 items=["White", "Black", "Inverted", "Black on White", "White on Black"] ("Color")
                w291 = i16 1 items=["Left", "Center", "Right"] ("Horizontal Alignment")
                # "灰度值小于20%的所有灰度值的平均值"
                # "GJB1038.A-2004缺陷评定时：\n人工缺陷检测面积A-缺陷实际面积W"
                # "0：位于蒙皮部位\n1：位于筋条部位"
                # "0 缺陷编号\n1 缺陷位置_X\n2 缺陷位置_Y\n3 缺陷长\n4 缺陷宽\n5 缺陷最大灰度值\n6 缺陷最小灰度值\n7 缺陷面积\n8 缺陷Z值\n9 缺陷位于哪个部位（0蒙皮，1筋条）\n10缺陷性质（1疏松类、2分层类，0其它轻微缺陷）\n11 缺陷合格性（0合格，1不合格）"
                # "确定测量"
                n140 = call "IMAQ GetImageSize"("Image"=w301) -> ("Y Resolution"=w307:i32, "X Resolution"=w306:i32)  [unwired: 3 in, 1 out]
                n141 = In Range and Coerce(upper limit=inf, x=w307, lower limit=w288) -> (In Range?=w309:bool)  [unwired: 1 out]
                n142 = In Range and Coerce(upper limit=inf, x=w306, lower limit=w288) -> (In Range?=w308:bool)  [unwired: 1 out]
                n143 = Select(t=w313, s=w314, f=w312) -> (s? t:f=w265:i32)
                n144 = Or(x=w309, y=w308) -> (x .or. y?=w287:bool)
                n145 = Select(t=i16 40 ("Size"), s=w287, f=i16 20) -> (s? t:f=w305:i16)
                n146 = call "任意角度矩形框尺寸计算及提取顶点坐标_子VI.vi"("Y向图像分辨率"=w299, "X向图像分辨率"=w300, "ROI Descriptor(任意角度矩形)"=w302) -> ("标准矩形框坐标（L、T、R、B）"=w283:i32[], "矩形宽（mm）"=w298:dbl, "矩形长（mm）"=w297:dbl, "矩形框各顶点坐标值"=w296:T15)  [unwired: 3 in, 2 out]
                n147 = call "IMAQ ImageToArray"("Optional Rectangle"=w283, "Image"=w301) -> ("Image Pixels (U8)"=w289:u8[][])  [unwired: 2 in, 4 out]
                n148 = for {
                  tunnel: w289 -> [w352] mode=indexing
                  tunnel: [w351] -> w326 mode=indexing
                  shift-right: [w349] -> w323
                  shift-left: 0.0 -> [w350]
                  n149 = for {
                    tunnel: w352 -> [w354] mode=indexing
                    tunnel: [w361] -> w351 mode=indexing
                    shift-right: [w355] -> w349
                    shift-left: w350 -> [w360]
                    n150 = To Double Precision Float(number=w354) -> (double precision float=w353:dbl)
                    n151 = Multiply(x=255.0, y=0.2) -> (x*y=w365:dbl)
                    n152 = Less?(x=w353, y=w365) -> (x < y?=w358:bool)
                    n153 = Select(t=1.0, s=w358, f=0.0) -> (s? t:f=w359:dbl)
                    n154 = Select(t=w353, s=w358, f=0.0) -> (s? t:f=w361:dbl)
                    n155 = Add(x=w360, y=w359) -> (x+y=w355:dbl)
                  }
                }
                n156 = Array Max & Min(array=w289) -> (max value=w327:u8, min value=w318:u8)  [unwired: 2 out]
                n157 = Index Array(array=w283, index #1=0 ("索引"), index #2=2 ("索引"), index #3=1 ("索引"), index #4=3 ("索引")) -> (element #1=w278:i32, element #2=w277:i32, element #3=w275:i32, element #4=w276:i32)
                n158 = Add(x=w278, y=w277) -> (x+y=w274:i32)
                n159 = Add(x=w275, y=w276) -> (x+y=w273:i32)
                n160 = Bundle By Name(cluster=T8 {"Font Name"="", "Size"=12, "Strikeout?"=FALSE, "Italic?"=FALSE, "Underline?"=FALSE, "Outline?"=FALSE, "Shadow?"=FALSE, "Bold?"=TRUE, "Rotation Angle"=0.0} ("[User-specified Font]"), "Size"=w305) -> (w343:T8)
                n161 = Unbundle By Name(w296) -> ("X右上"=w286:i32, "Y右上"=w285:i32)
                n162 = Divide(x=w274, y=w272) -> (x/y=w271:dbl)
                n163 = Divide(x=w273, y=w272) -> (x/y=w270:dbl)
                n164 = call "任意角度矩形框绘制_子VI.vi"("任意角度矩形框各顶点坐标值"=w296, "Image"=w301) -> ("Image Out"=w284:T3)  [unwired: 9 in]
                n165 = Bundle By Name(cluster=T9 {"Desired Font (Application)"=enum."User-specified Font", "[User-specified Font]"={"Font Name"="", "Size"=12, "Strikeout?"=FALSE, "Italic?"=FALSE, "Underline?"=TRUE, "Outline?"=FALSE, "Shadow?"=FALSE, "Bold?"=TRUE, "Rotation Angle"=0.0}, "Horizontal Alignment"=0, "Vertical Alignment"=0} ("Font, Size & Style"), "[User-specified Font]"=w343, "Horizontal Alignment"=w291, "Vertical Alignment"=w290) -> (w344:T9)
                n166 = Round To Nearest(number=w271) -> (nearest integer value=w268:dbl)
                n167 = Round To Nearest(number=w270) -> (nearest integer value=w269:dbl)
                n168 = Build Array(w286, w285) -> (w347:i32[])
                n169 = Increment(x=w292) -> (x+1=w267:i32)
                n170 = Add Array Elements(numeric array=w326) -> (sum=w320:dbl)
                n171 = Equal To 0?(x=w323) -> (x = 0?=w321:bool)
                n172 = To Double Precision Float(number=w318) -> (double precision float=w319:dbl)
                n173 = Number To Decimal String(number=w267) -> (decimal integer string=w295:string)  [unwired: 1 in]
                n174 = Select(t=1.0, s=w321, f=w323) -> (s? t:f=w322:dbl)
                n175 = Select(t=w319, s=w321, f=w320) -> (s? t:f=w317:dbl)
                n176 = Concatenate Strings(w295, "#" ("字符串")) -> (w293:string)
                n177 = call "缺陷部位标注"() -> ("位于筋条处"=w334:bool, "位于蒙皮处"=w335:bool)  [unwired: 16 in, 2 out]
                n178 = Divide(x=w317, y=w322) -> (x/y=w316:dbl)
                n179 = call "IMAQ Draw Text"("String"=w293, "Insertion Point"=w347, "Color"=w265, "Font, Size & Style"=w344, "Image Dst"=w284, "Image Src"=w284) -> ("Image Dst Out"=w346:T3)  [unwired: 2 in, 3 out]
                n180 = To Unsigned Byte Integer(number=w316) -> (unsigned 8bit integer=w315:u8)
                n181 = Build Array(w335, w334) -> (w333:bool[])
                n182 = local write "Image"(w346) -> ()
                n183 = Boolean Array To Number(Boolean array=w333) -> (number=w332:u32)
                n184 = Multiply(x=w297, y=w298) -> (x*y=w330:dbl)
                n185 = case shown="1, 默认" w332 {
                  tunnel: [0.0 ("t") 1.0 ("t")] -> w331
                  frame 1, Default {
                  }
                  frame 2 {
                  }
                }
                n186 = Subtract(x=w330, y=w328) -> (x-y=w329:dbl)
                n187 = Add(x=w297, y=w298) -> (x+y=w337:dbl)
                n188 = Increment(x=w292) -> (x+1=w266:i32)
                n189 = Divide(x=w337, y=2.0) -> (x/y=w338:dbl)
                n190 = Build Array(w266, w268, w269, w297, w298, w327, w315, w329, w338, w331, w336, w336) -> (w341:dbl[])
                n191 = Increment(x=w292) -> (x+1=w348:i32)
                n192 = Replace Array Subset(array=w342, new element=w341, index (row)=w292) -> (w340:dbl[][])  [unwired: 1 in]
              }
              frame True {
                # "取消测量，维持原数据"
              }
            }
          }
          frame Error {
          }
        }
        n193 = Current VI's Path() -> (path=w243:path)
        n194 = Open VI Reference(vi path=w243, error in (no error)=w226) -> (vi reference=w242:refnum<vi>, error out=w239:errorcluster)  [unwired: 4 in]
        n195 = property class="VI"(reference=w242, error in=w239, "FP.State"=T5."Standard" ("前面板窗口:状态")) -> (reference out=w240:refnum<vi>, error out=w238:errorcluster)
        n196 = Close Reference(reference=w240, error in (no error)=w238) -> ()  [unwired: 1 out]
      }
      event "缺陷分析及评定": Value Change {
        # "人工辅助判断缺陷性质\n定性依据：\n1、（最小灰度值/255）≤20%且缺陷位于蒙皮部位，认定为疏松类缺陷；\n2、（最小灰度值/255）≤20%且缺陷位于筋条部位，疑似分层缺陷，弹出提示框，由人工采用辅助试验进行定性；\n3、（最小灰度值/255）>30%，认定为不明显缺陷。\n\n合格判据：\n1、疏松类缺陷计算缺陷面积占评定面积的百分比，分层缺陷计算Z值；\n2、缺陷面积或Z值不满足GJB2895 B级（或更改后的级别）要求时判定为不合格。"
        n197 = event-data() -> ()  [unwired: 1 in, 6 out]
        n198 = flat-sequence {
          tunnel: [w400] -> w385
          tunnel: [w399] -> w384
          tunnel: [w398] -> w383
          tunnel: w385 -> [w405]
          tunnel: w384 -> [w404]
          tunnel: [w402] -> w382
          frame #0 {
            w399 = "复材分析评定软件" ("section")
            w400 = "判定阈值配置" ("文件名称")
            n199 = call-poly "ini配置文件读取.vi"("key"="Z值", "section"=w399, "文件名称"=w400) -> ("value"=w398:dbl)  [unwired: 8 in]
          }
          frame #1 {
            n200 = call-poly "ini配置文件读取.vi"("key"="弥散性缺陷阈值", "section"=w404, "文件名称"=w405) -> ("value"=w402:dbl)  [unwired: 8 in]
          }
        }
        n201 = Two Button Dialog(message="是否进行缺陷分析评定？\n分析前请确认已进行缺陷测量！" ("消息")) -> (T button?=w386:bool)  [unwired: 2 in]
        n202 = case shown="真" w386 {
          tunnel: w396 -> [w406 w425]
          tunnel: [w406 w412] -> w395
          tunnel: [_ errorcluster {"status"=FALSE, "code"=0, "source"=""} ("错误常量")] -> w387
          tunnel: w383 -> [_ w410]
          tunnel: w382 -> [_ w409]
          frame False {
          }
          frame True {
            w414 = 0.0
            # "将合格性结果输出，并填入缺陷信息数组中（第11列）"
            # "缺陷Z值"
            # "疑似分层数量"
            # "将定性结果输出，并填入缺陷信息数组中（第10列）"
            # "0 缺陷编号\n1 缺陷位置_X\n2 缺陷位置_Y\n3 缺陷长\n4 缺陷宽\n5 缺陷最大灰度值\n6 缺陷最小平均灰度值\n7 缺陷面积\n8 缺陷Z值\n9 缺陷位于哪个部位（0蒙皮，1筋条）\n10缺陷性质（1疏松类、2疑似分层类，0其它轻微缺陷）\n11 缺陷合格性（0合格，1不合格）"
            n203 = Index Array(array=w425, index (col) #1=8 ("禁用的索引 (列)"), index (col) #2=7 ("禁用的索引 (列)"), index (col) #3=6 ("禁用的索引 (列)"), index (col) #4=9 ("索引 (列)"), index (col) #5=0 ("索引 (列)")) -> (element #1=w419:dbl[], element #2=w418:dbl[], element #3=w432:dbl[], element #4=w430:dbl[], element #5=w423:dbl[])  [unwired: 5 in]
            n204 = Array Max & Min(array=w423) -> (max value=w407:dbl)  [unwired: 3 out]
            n205 = for {
              N: w407 -> [_]
              tunnel: w432 -> [w490] mode=indexing
              tunnel: w430 -> [w486] mode=indexing
              tunnel: [w464] -> w428 mode=indexing
              shift-right: [w473] -> w427
              shift-left: w414 -> [w474]
              shift-right: [w467] -> w426
              shift-left: w414 -> [w468]
              tunnel: w419 -> [w463] mode=indexing
              tunnel: w418 -> [w462] mode=indexing
              tunnel: [w460] -> w415 mode=indexing
              shift-right: [w461] -> w413
              shift-left: w414 -> [w459]
              tunnel: w410 -> [w458]
              tunnel: w409 -> [w457]
              # "缺陷面积"
              # "疑似分层缺陷"
              # "疏松类缺陷"
              n206 = Equal?(x=w486, y=0.0) -> (x = y?=w484:bool)
              n207 = Divide(x=w490, y=255.0) -> (x/y=w488:dbl)
              n208 = Select(t=1.0, s=w484, f=2.0) -> (s? t:f=w481:dbl)
              n209 = Less Or Equal?(x=w488, y=0.3) -> (x <= y?=w472:bool)
              n210 = Select(t=w481, s=w472, f=0.0) -> (s? t:f=w464:dbl)
              n211 = case shown="1" w464 {
                tunnel: w463 -> [_ _ w509]
                tunnel: w462 -> [_ w499 _]
                tunnel: [0.0 ("f") w493 w510] -> w460
                tunnel: w458 -> [_ _ w508]
                tunnel: w457 -> [_ w492 _]
                frame 0, Default {
                  # "其它缺陷"
                }
                frame 1 {
                  (unwired) 0.15 ("y")
                  # "疏松类缺陷"
                  n212 = local read "产品规格"() -> (w507:cluster{"产品长度（周长）（mm）":dbl, "产品宽度（母线长）（mm）":dbl})
                  n213 = Unbundle(w507) -> ("产品长度（周长）（mm）"=w505:dbl, "产品宽度（母线长）（mm）"=w506:dbl)
                  n214 = Divide(x=w505, y=w506) -> (x/y=w504:dbl)
                  n215 = Greater Or Equal?(x=w504, y=10.0) -> (x >= y?=w502:bool)
                  n216 = Select(t=6400.0, s=w502, f=15500.0) -> (s? t:f=w498:dbl)
                  n217 = Divide(x=w499, y=w498) -> (x/y=w497:dbl)
                  n218 = Greater?(x=w497, y=w492) -> (0:w496:bool)
                  n219 = Select(t=1.0, s=w496, f=0.0) -> (s? t:f=w493:dbl)
                }
                frame 2 {
                  (unwired) 13.0 ("y")
                  # "疑似分层类缺陷"
                  n220 = Greater?(x=w509, y=w508) -> (0:w513:bool)
                  n221 = Select(t=1.0, s=w513, f=0.0) -> (s? t:f=w510:dbl)
                }
              }
              n222 = Equal?(x=w464, y=1.0 ("x")) -> (x = y?=w465:bool)
              n223 = Select(t=1.0, s=w465, f=0.0) -> (s? t:f=w469:dbl)
              n224 = Add(x=w469, y=w468) -> (x+y=w467:dbl)
              n225 = Equal?(x=2.0, y=w464) -> (x = y?=w478:bool)
              n226 = Select(t=1.0, s=w478, f=0.0) -> (s? t:f=w475:dbl)
              n227 = Add(x=w474, y=w475) -> (x+y=w473:dbl)
              n228 = Add(x=w459, y=w460) -> (x+y=w461:dbl)
            }
            n229 = Replace Array Subset(array=w425, new element=w428, index (col)=10 ("禁用的索引 (列)")) -> (w416:dbl[][])  [unwired: 1 in]
            n230 = Replace Array Subset(array=w416, new element=w415, index (col)=11 ("禁用的索引 (列)")) -> (w412:dbl[][])  [unwired: 1 in]
            n231 = flat-sequence {
              tunnel: [w434] -> w408
              frame #0 {
                n232 = Current VI's Path() -> (path=w440:path)
                n233 = Open VI Reference(vi path=w440) -> (vi reference=w439:refnum<vi>, error out=w436:errorcluster)  [unwired: 5 in]
                n234 = property class="VI"(reference=w439, error in=w436, "FP.State"=T5."Hidden" ("前面板窗口:状态")) -> (reference out=w437:refnum<vi>, error out=w435:errorcluster)
                n235 = Close Reference(reference=w437, error in (no error)=w435) -> (error out=w434:errorcluster)
              }
            }
            n236 = for {
              N: w407 -> [_]
              tunnel: w412 -> [w441] mode=indexing
              tunnel: [w441] -> w422 mode=indexing
            }
            n237 = case shown="无错误" w408 {
              tunnel: w422 -> [w443 _]
              tunnel: w427 -> [w445 _]
              tunnel: w426 -> [w446 _]
              tunnel: w407 -> [w448 _]
              tunnel: w413 -> [w444 _]
              frame No Error {
                # "评定结果显示"
                n238 = Subtract(x=w448, y=w445) -> (x-y=w449:dbl)
                n239 = Subtract(x=w449, y=w446) -> (x-y=w447:dbl)
                n240 = Bundle(w444, w448, w447, w446, w445, w443) -> (w442:cluster{dbl, dbl, dbl, dbl, dbl, dbl[][]})  [unwired: 1 in]
                "辅助缺陷评定结果" <- w442
                n241 = flat-sequence {
                  tunnel: w442 -> [w456]
                  frame #0 {
                    n242 = Unbundle(w456) -> (w455:dbl, w454:dbl, w453:dbl, w452:dbl, w451:dbl, w450:dbl[][])
                    n243 = call "缺陷评定结果显示子VI.vi"("疑似分层类缺陷数"=w451, "不合格缺陷数"=w455, "疏松类缺陷数"=w452, "其它缺陷数"=w453, "总缺陷数"=w454, "评定结果"=w450) -> ()  [unwired: 5 in, 1 out]
                  }
                }
              }
              frame Error {
              }
            }
          }
        }
        n244 = Current VI's Path() -> (path=w393:path)
        n245 = Open VI Reference(vi path=w393, error in (no error)=w387) -> (vi reference=w392:refnum<vi>, error out=w389:errorcluster)  [unwired: 4 in]
        n246 = property class="VI"(reference=w392, error in=w389, "FP.State"=T5."Standard" ("前面板窗口:状态")) -> (reference out=w390:refnum<vi>, error out=w388:errorcluster)
        n247 = Close Reference(reference=w390, error in (no error)=w388) -> ()  [unwired: 1 out]
      }
      event "去除标注信息": Value Change {
        # "去除所有标注信息，并恢复为原图"
        n248 = event-data() -> ()  [unwired: 1 in, 6 out]
        n249 = local read "Source Image Pixels (U8)"() -> (w520:u8[][])
        n250 = call "IMAQ Create"("Image Name"="P2") -> ("New Image"=w521:T3)  [unwired: 4 in, 1 out]
        n251 = call "IMAQ ArrayToImage"("Image Pixels (U8)"=w520, "Image"=w521) -> ("Image Out"=w522:T3)  [unwired: 8 in, 1 out]
        n252 = local write "Image"(w522) -> ()
        n253 = Initialize Array(0.0 ("元素"), 300 ("维数大小"), 12 ("维数大小")) -> (w515:dbl[][])
      }
      event "生成原始记录": Value Change {
        # "0 缺陷编号\n1 缺陷位置_X\n2 缺陷位置_Y\n3 缺陷长\n4 缺陷宽\n5 缺陷最大灰度值\n6 缺陷最小灰度值\n7 缺陷面积\n8 缺陷Z值\n9 缺陷位于哪个部位（0蒙皮，1筋条）\n10缺陷性质（1疏松类、2分层类，0其它轻微缺陷）\n11 缺陷合格性（0合格，1不合格）"
        # "按格式生成原始记录"
        n254 = event-data() -> ()  [unwired: 1 in, 6 out]
        n255 = flat-sequence {
          tunnel: [w570] -> w525
          tunnel: [w569] -> w524
          tunnel: [w568] -> w523
          frame #0 {
            n256 = local read "Image Path"() -> (w569:path)
            n257 = Path To String(path=w569) -> (string=w575:string)
            n258 = String Length(string=w575) -> (length=w574:i32)
            n259 = Subtract(x=w574, y=4) -> (x-y=w573:i32)
            n260 = Replace Substring(3:w573, 4:"_标注后.png" ("字符串"), 5:w575) -> (1:w580:string)  [unwired: 1 in, 1 out]
            n261 = property on="Image" class="ImageControl"() -> ("Palette Type"=w579:u32)  [unwired: 2 in, 2 out]
            n262 = String To Path(string=w580) -> (path=w570:path)
            n263 = case shown="0, 默认" w579 {
              tunnel: [w581 w583 w585 w587 w589] -> w578
              frame 0, Default {
                # "灰度"
                n264 = call "IMAQ GetPalette"("Palette Number (gray)"=T7."Gray") -> ("Color Palette"=w581:cluster{"Red":u8, "Green":u8, "Blue":u8}[])  [unwired: 4 in, 1 out]
              }
              frame 2 {
                # "梯度"
                n265 = call "IMAQ GetPalette"("Palette Number (gray)"=T7."Gradient") -> ("Color Palette"=w583:cluster{"Red":u8, "Green":u8, "Blue":u8}[])  [unwired: 4 in, 1 out]
              }
              frame 3 {
                # "彩虹"
                n266 = call "IMAQ GetPalette"("Palette Number (gray)"=T7."Rainbow") -> ("Color Palette"=w585:cluster{"Red":u8, "Green":u8, "Blue":u8}[])  [unwired: 4 in, 1 out]
              }
              frame 4 {
                # "温度"
                n267 = call "IMAQ GetPalette"("Palette Number (gray)"=T7."Temperature") -> ("Color Palette"=w587:cluster{"Red":u8, "Green":u8, "Blue":u8}[])  [unwired: 4 in, 1 out]
              }
              frame 5 {
                # "自定义"
                n268 = property on="Image" class="ImageControl"() -> ("User Palette"=w589:cluster{"Red":u8, "Green":u8, "Blue":u8}[])  [unwired: 2 in, 2 out]
              }
            }
            n269 = local read "Image"() -> (w577:T3)
            n270 = call-poly "IMAQ Write File 2"("Color Palette"=w578, "Image Quality"=u32 1000, "File Path"=w570, "Image"=w577) -> ("error out"=w568:errorcluster)  [unwired: 6 in, 1 out]
          }
        }
        n271 = local read "辅助缺陷评定结果"() -> (w529:cluster{dbl, dbl, dbl, dbl, dbl, dbl[][]})
        n272 = Unbundle(w529) -> (w528:dbl[][])  [unwired: 5 out]
        n273 = Index Array(array=w528, index (col) #1=0 ("禁用的索引 (列)"), index (col) #2=1 ("索引 (列)"), index (col) #3=2 ("索引 (列)"), index (col) #4=3 ("索引 (列)"), index (col) #5=4 ("索引 (列)"), index (col) #6=5 ("索引 (列)"), index (col) #7=6 ("索引 (列)"), index (col) #8=7 ("索引 (列)"), index (col) #9=8 ("索引 (列)"), index (col) #10=9 ("索引 (列)"), index (col) #11=10 ("索引 (列)"), index (col) #12=11 ("索引 (列)")) -> (element #1=w554:dbl[], element #2=w553:dbl[], element #3=w552:dbl[], element #4=w551:dbl[], element #5=w550:dbl[], element #6=w549:dbl[], element #7=w548:dbl[], element #8=w547:dbl[], element #9=w546:dbl[], element #10=w545:dbl[], element #11=w544:dbl[], element #12=w543:dbl[])  [unwired: 12 in]
        n274 = for {
          tunnel: w554 -> [w658] mode=indexing
          tunnel: w553 -> [w657] mode=indexing
          tunnel: w552 -> [w656] mode=indexing
          tunnel: w551 -> [w655] mode=indexing
          tunnel: w550 -> [w654] mode=indexing
          tunnel: w549 -> [w653] mode=indexing
          tunnel: w548 -> [w652] mode=indexing
          tunnel: w547 -> [w651] mode=indexing
          tunnel: w546 -> [w650] mode=indexing
          tunnel: w545 -> [w648] mode=indexing
          tunnel: w544 -> [w647] mode=indexing
          tunnel: w543 -> [w646] mode=indexing
          tunnel: [w632] -> w542 mode=indexing
          tunnel: [w645] -> w541 mode=indexing
          tunnel: [w644] -> w540 mode=indexing
          tunnel: [w643] -> w539 mode=indexing
          tunnel: [w642] -> w538 mode=indexing
          tunnel: [w641] -> w537 mode=indexing
          tunnel: [w640] -> w536 mode=indexing
          tunnel: [w639] -> w535 mode=indexing
          tunnel: [w638] -> w534 mode=indexing
          tunnel: [w637] -> w533 mode=indexing
          tunnel: [w636] -> w531 mode=indexing
          tunnel: [w635] -> w532 mode=indexing
          w649 = i16 1 ("精度(6)")
          n275 = case shown="0, 默认" w648 {
            tunnel: ["蒙皮处" "筋条处"] -> w637
            frame 0, Default {
            }
            frame 1 {
            }
          }
          n276 = case shown="1" w647 {
            tunnel: ["其他轻微缺陷" "疏松类" "疑似分层类"] -> w635
            frame 0, Default {
            }
            frame 1 {
            }
            frame 2 {
            }
          }
          n277 = case shown="1" w646 {
            tunnel: ["合格" "不合格"] -> w636
            frame 0, Default {
            }
            frame 1 {
            }
          }
          n278 = Number To Decimal String "数值至十进制数字符串转换"(number=w658) -> (decimal integer string=w634:string)  [unwired: 1 in]
          n279 = Number To Fractional String(number=w657, precision (6)=w649) -> (F-format string=w645:string)  [unwired: 2 in]
          n280 = Number To Fractional String(number=w656, precision (6)=w649) -> (F-format string=w644:string)  [unwired: 2 in]
          n281 = Number To Fractional String(number=w655, precision (6)=w649) -> (F-format string=w643:string)  [unwired: 2 in]
          n282 = Number To Fractional String(number=w654, precision (6)=w649) -> (F-format string=w642:string)  [unwired: 2 in]
          n283 = Number To Fractional String(number=w653, precision (6)=w649) -> (F-format string=w641:string)  [unwired: 2 in]
          n284 = Number To Fractional String(number=w652, precision (6)=w649) -> (F-format string=w640:string)  [unwired: 2 in]
          n285 = Number To Fractional String(number=w651, precision (6)=w649) -> (F-format string=w639:string)  [unwired: 2 in]
          n286 = Number To Fractional String(number=w650, precision (6)=w649) -> (F-format string=w638:string)  [unwired: 2 in]
          n287 = Concatenate Strings(w634, "#" ("字符串")) -> (w632:string)
        }
        n288 = Build Array(w542, w541, w540, w539, w538, w537, w536, w535, w534, w533, w532, w531) -> (w530:string[][])
        n289 = Transpose 2D Array(2D array=w530) -> (transposed array=w526:string[][])
        n290 = case shown="无错误" w523 {
          tunnel: w526 -> [w609 _]
          tunnel: w525 -> [w591 _]
          tunnel: w524 -> [w590 _]
          frame No Error {
            n291 = call "路径处理子VI.vi"("文件名称（包括后缀）"="report-template.docx" ("名称或相对路径")) -> ("添加的路径"=w593:path)  [unwired: 10 in]
            n292 = Format Date/Time String(time format string (%c)="%y%m%d" ("时间格式字符串(%c)")) -> (date/time string=w600:string)  [unwired: 2 in]
            n293 = Strip Path(path=w590) -> (stripped path=w598:path, name=w606:string)
            n294 = String Length(string=w606) -> (length=w608:i32)
            n295 = Subtract(x=w608, y=4) -> (x-y=w605:i32)
            n296 = Concatenate Strings("__缺陷分析评定记录" ("子字符串(\"\")"), w600, ".docx" ("字符串")) -> (w604:string)
            n297 = Replace Substring(3:w605, 4:w604, 5:w606) -> (1:w599:string)  [unwired: 1 in, 1 out]
            n298 = call "产品名称及编号"() -> ("产品名称编号"=w596:string, "确定"=w595:bool)  [unwired: 17 in, 1 out]
            n299 = Build Path(base path=w598, name or relative path=w599) -> (appended path=w597:path)
            n300 = case shown="真" w595 {
              tunnel: w609 -> [_ w631]
              tunnel: w593 -> [_ w630]
              tunnel: errorcluster {"status"=FALSE, "code"=0, "source"=""} ("error in (no error)") -> [_ w629]
              tunnel: w591 -> [_ w628]
              tunnel: w597 -> [_ w627]
              tunnel: w596 -> [_ w626]
              frame False {
              }
              frame True {
                w618 = "\r"
                n301 = call-poly "ini配置文件读取.vi"("key"="office", "section"="复材分析评定软件", "文件名称"="判定阈值配置") -> ("value"=w614:dbl)  [unwired: 8 in]
                n302 = Equal To 0?(x=w614) -> (x = 0?=w613:bool)
                n303 = Select(t=10.0, s=w613, f=0.65 ("column width (1)")) -> (s? t:f=w610:dbl)
                n304 = call "报告生成子VI.vi"("column width (1)"=w610, "error in (no error)"=w629, "产品编号"=w626, "text data"=w631, "报告保存路径"=w627, "标注后的图片路径"=w628, "报告模板路径"=w630) -> ("报告存储路径"=w623:path, "标注后的图片存储路径"=w625:path)  [unwired: 3 in]
                n305 = Path To String(path=w625) -> (string=w624:string)
                n306 = Path To String(path=w623) -> (string=w620:string)
                n307 = Concatenate Strings("图片已保存在：" ("string"), w618, w624, w618, w618, "原始记录已保存在：" ("string"), w618, w620) -> (w622:string)
                n308 = One Button Dialog(message=w622) -> ()  [unwired: 1 in, 1 out]
              }
            }
          }
          frame Error {
          }
        }
      }
      event "stop": Value Change {
        # "退出软件"
        n309 = event-data() -> ("NewVal"=w669:bool)  [unwired: 1 in, 4 out]
        n310 = Two Button Dialog(message="是否关闭本软件？" ("消息")) -> (T button?=w671:bool)  [unwired: 2 in]
        n311 = And(x=w669, y=w671) -> (x .and. y?=w668:bool)
        n312 = case shown="真" w668 {
          frame False {
          }
          frame True {
            n313 = local read "Image"() -> (w673:T3)
            n314 = call "IMAQ Dispose"("All Images? (No)"=TRUE, "Image"=w673) -> ()  [unwired: 4 in, 1 out]
            n315 = disable-structure shown="RUN_TIME_ENGINE==True" {
              frame condition #0 {
                n316 = Quit LabVIEW() -> ()  [unwired: 1 in]
              }
              frame condition #1 (active) {
                n317 = Stop() -> ()  [unwired: 1 in]
              }
            }
          }
        }
      }
    }
  }
